vi "RainbowAnimation SetControl.vi"(0 "DeviceReference":T1, 7 "error in":errorcluster, 18 "Update Frequency (Hz)":dbl=100.0) -> (20 "DeviceReference Out":T1, 27 "error out":errorcluster)   [LabVIEW 2025]
uses:
  <vilib>/Rock Robotics/WPI/ThirdParty/Phoenix6/DeviceReference.ctl
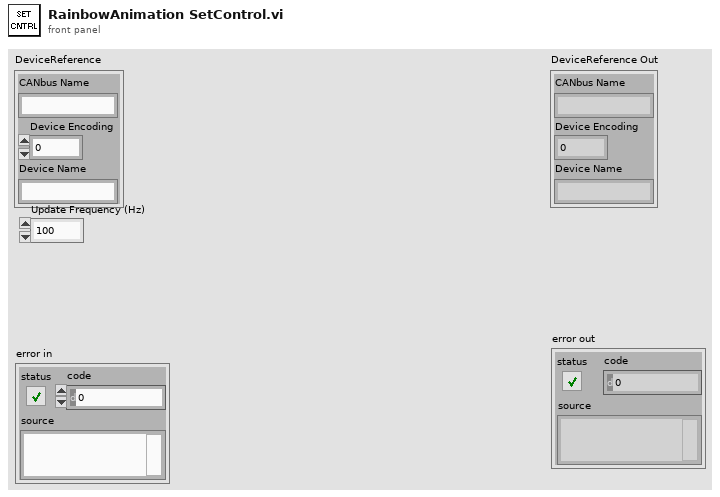
[diagram p1: front panel]
types:
  T1 = typedef "DeviceReference.ctl" = cluster{"CANbus Name":string, "Device Encoding":u32, "Device Name":string}
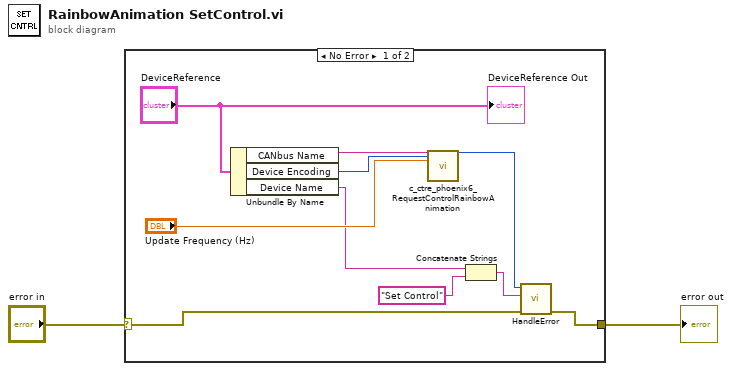
[diagram p0: block diagram]
diagram:
  n1 = case shown="No Error" "error in" {
    selector: "error in" -> [w7 w13]
    tunnel: [w6 w13] -> w1
    frame No Error {
      n2 = Unbundle By Name("DeviceReference") -> ("CANbus Name"=w11:string, "Device Encoding"=w10:u32, "Device Name"=w5:string)
      n3 = call <vilib>:"c_ctre_phoenix6_RequestControlRainbowAnimation.vi"("String 2"=w11, "Numeric 2"=w10, "Numeric 3"="Update Frequency (Hz)") -> ("Numeric"=w8:i32)  [unwired: 23 in, 1 out]
      n4 = Concatenate Strings(w5, "Set Control" ("origin")) -> (w3:string)
      n5 = call <vilib>:"HandleError.vi"("error in"=w7, "origin"=w3, "Status"=w8) -> ("error out"=w6:errorcluster)  [unwired: 8 in]
      "DeviceReference Out" <- "DeviceReference"
    }
    frame Error {
    }
  }
  "error out" <- w1
